vi "Initialize Instrument.vi"(8 "error in (no error)":errorcluster, 10 "Instr Resource Str":string, 11 "Simulated Sig Gen.lvclass in":refnum<class "Simulated Sig Gen.lvclass">) -> (0 "error out":errorcluster, 3 "Simulated Sig Gen.lvclass out":refnum<class "Simulated Sig Gen.lvclass">)   [LabVIEW 2010, in "Simulated Sig Gen.lvclass"]
uses:
  Simulated Sig Gen.lvclass
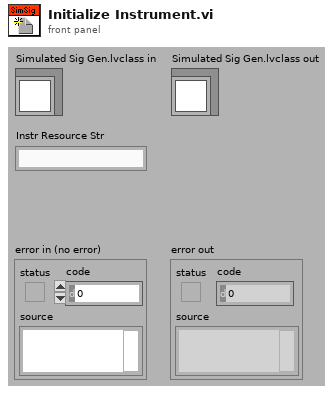
[diagram p1: front panel]
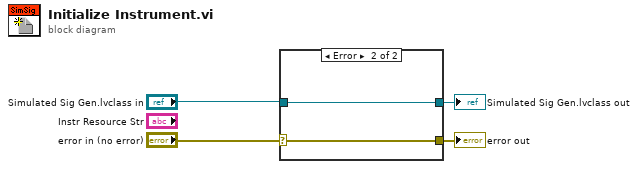
[diagram p0: block diagram]
diagram:
  n1 = case shown="Error" "error in (no error)" {
    selector: "error in (no error)" -> [w5 w8]
    tunnel: [w5 w8] -> w4
    tunnel: "Simulated Sig Gen.lvclass in" -> [w6 w7]
    tunnel: [w6 w7] -> w3
    frame No Error {
    }
    frame Error {
    }
  }
  "error out" <- w4
  "Simulated Sig Gen.lvclass out" <- w3
